vi "Constants.vi"() -> ()   [LabVIEW 2019]
panel:
  in  "Track Width":dbl=25.0
  in  "CenterRotOffset":dbl=17.0
  in  "Length":dbl=38.5
  in  "Width":dbl=31.5
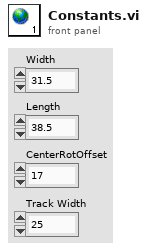
[diagram p1: front panel]
diagram:
